vi "[Top Level] Multi Listbox.vi"() -> ()   [LabVIEW 2012]
uses:
  <vilib>/Utility/miscctls.llb/LVPoint32TypeDef.ctl
  <vilib>/Utility/error.llb/DialogType.ctl
  Method/Get Cell Item From Index.vi
  Mlistbox Tools.lvlib
panel:
  in  "Popup Listbox":i32(listbox)=4
  out "Multicolumn Listbox":i32(listbox)
  in  "Stop":bool
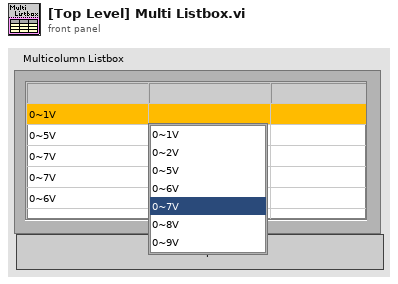
[diagram p1: front panel]
types:
  T1 = typedef "LVPoint32TypeDef.ctl" = cluster{"Horizontal":i32, "Vertical":i32}
  T2 = cluster{"State":enum16{"Initialize Multi Listbox", "Get Active Cell", "Get ItemName", "Set Symbol", "Set ItemName", "IDLE", "Error", "Exit"}, "Data":variant}
  T3 = cluster{"Multicolumn Listbox":refnum<vi>, "Popup Listbox":refnum<vi>, "Coords":T1, "Active Cell":cluster{"Row":i32, "Column":i32}, "Visible?":bool, "ItemName":string}
  T4 = enum16{"Initialize Multi Listbox", "Get Active Cell", "Get ItemName", "Set Symbol", "Set ItemName", "IDLE", "Error", "Exit"}
  T5 = cluster{"State":enum16{"Initialize Multi Listbox", "Get Active Cell", "Get ItemName", "Set Symbol", "Set ItemName", "IDLE", "Error", "Exit"}, "Data":variant}[]
  T6 = typedef "LVRowAndColumnTypeDef.ctl" = cluster{"Row":i32, "Column":i32}
  T7 = typedef "DialogType.ctl" = u16
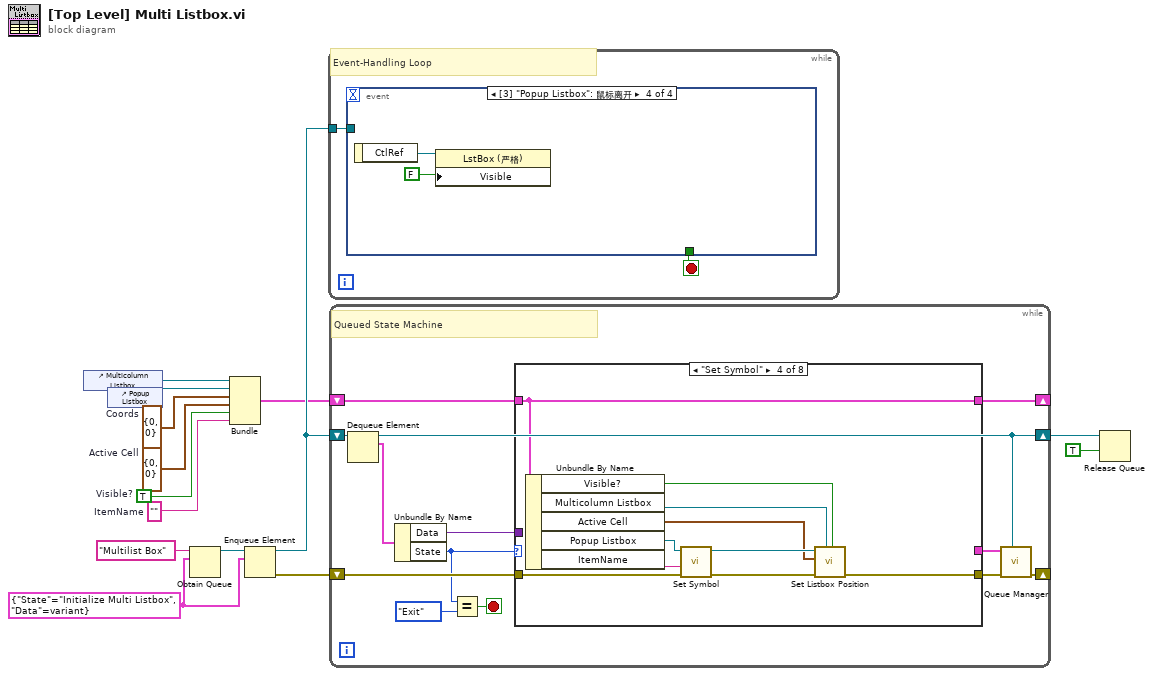
[diagram p0: block diagram]
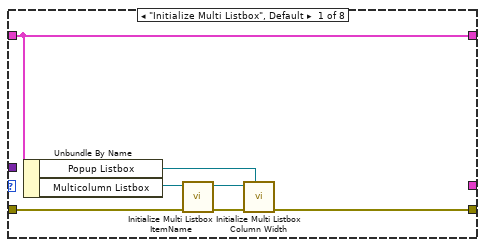
[diagram p2: hidden frame]
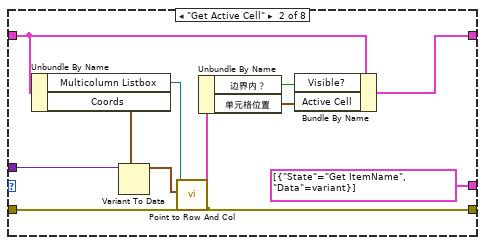
[diagram p3: hidden frame]
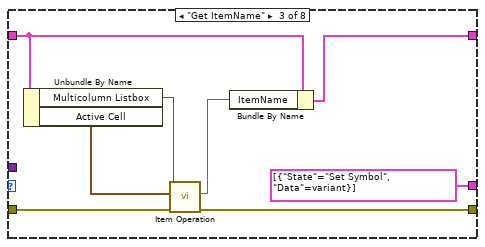
[diagram p4: hidden frame]
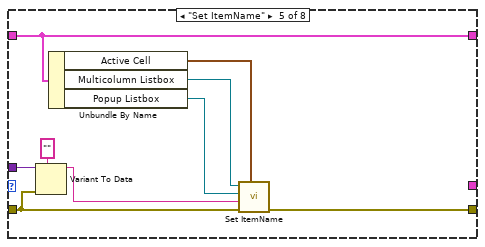
[diagram p5: hidden frame]
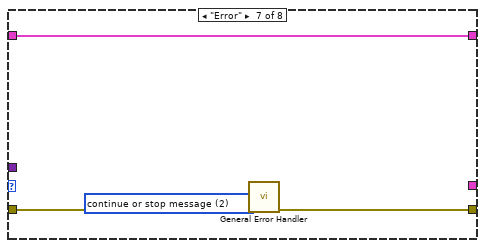
[diagram p7: hidden frame]
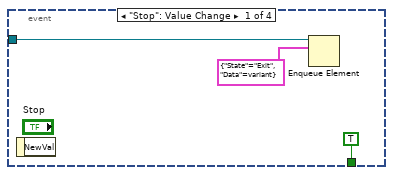
[diagram p9: hidden frame]
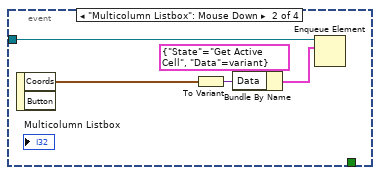
[diagram p10: hidden frame]
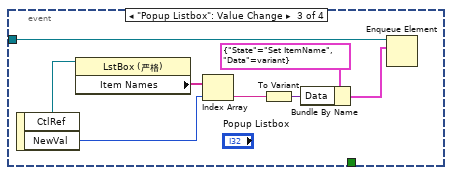
[diagram p11: hidden frame]
diagram:
  w1 = ""  # ItemName
  w2 = TRUE  # Visible?
  w3 = cluster{"Row":i32, "Column":i32} {"Row"=0, "Column"=0}  # Active Cell
  w4 = T1 {"Horizontal"=0, "Vertical"=0}  # Coords
  w8 = T2 {"State"=enum."Initialize Multi Listbox", "Data"=variant} ("Element")
  n1 = control-ref of="Multicolumn Listbox"() -> (w7:refnum<vi>)
  n2 = control-ref of="Popup Listbox"() -> (w6:refnum<vi>)
  n3 = Obtain Queue(name (unnamed)="Multilist Box", element data type=w8) -> (queue out=w10:refnum<queue>)  [unwired: 3 in, 2 out]
  n4 = Bundle ("捆绑")("Multicolumn Listbox"=w7, "Popup Listbox"=w6, "Coords"=w4, "Active Cell"=w3, "Visible?"=w2, "ItemName"=w1) -> (w5:T3)  [unwired: 1 out]
  n5 = Enqueue Element(queue=w10, element=w8) -> (queue out=w14:refnum<queue>, error out=w11:errorcluster)  [unwired: 1 in, 2 out]
  n6 = while {
    tunnel: w14 -> [w16]
    stop <- w15 stop-if-true
    # "Event-Handling Loop"
    n7 = event shown="[3] \"Popup Listbox\": 鼠标离开" {
      selector: _ -> [_ _ _ _]
      dyn-events: _ -> [_ _ _ _]
      timeout: _ -> [_ _ _ _]
      tunnel: w16 -> [w19 w24 w32 _]
      tunnel: [TRUE _ _ _] -> w15
      event "Stop": Value Change {
        n8 = event-data() -> ()  [unwired: 2 out]
        n9 = Enqueue Element(queue=w19, element=T2 {"State"=enum."Exit", "Data"=variant}) -> ()  [unwired: 1 in, 4 out]
      }
      event "Multicolumn Listbox": Mouse Down {
        n10 = event-data() -> ("Coords"=w20:T1)  [unwired: 2 out]
        n11 = To Variant(anything=w20) -> (Variant=w21:variant)
        n12 = Bundle By Name(cluster=T2 {"State"=enum."Get Active Cell", "Data"=variant} ("element"), "Data"=w21) -> (w22:T2)
        n13 = Enqueue Element(queue=w24, element=w22) -> ()  [unwired: 1 in, 4 out]
      }
      event "Popup Listbox": Value Change {
        n14 = event-data() -> ("CtlRef"=w28:refnum<vi>, "NewVal"=w26:i32)  [unwired: 1 out]
        n15 = property class="LstBox (严格)"(reference=w28) -> ("Item Names"=w27:string[])  [unwired: 1 in, 2 out]
        n16 = Index Array(array=w27, index=w26) -> (element=w25:string)
        n17 = To Variant(anything=w25) -> (Variant=w29:variant)
        n18 = Bundle By Name(cluster=T2 {"State"=enum."Set ItemName", "Data"=variant} ("element"), "Data"=w29) -> (w30:T2)
        n19 = Enqueue Element(queue=w32, element=w30) -> ()  [unwired: 1 in, 4 out]
      }
      event "Popup Listbox": Mouse Leave {
        n20 = event-data() -> ("CtlRef"=w34:refnum<vi>)  [unwired: 1 out]
        n21 = property class="LstBox (严格)"(reference=w34, "Visible"=FALSE) -> ()  [unwired: 1 in, 2 out]
      }
    }
  }
  n22 = while {
    shift-right: [w40] -> _
    shift-left: w11 -> [w44]
    shift-right: [w41] -> w12
    shift-left: w14 -> [w47]
    shift-right: [w37] -> _
    shift-left: w5 -> [w38]
    stop <- w42 stop-if-true
    # "Queued State Machine"
    n23 = Dequeue Element(queue=w47) -> (queue out=w41:refnum<queue>, element=w46:T2)  [unwired: 1 in, 3 out]
    n24 = Unbundle By Name(w46) -> ("Data"=w45:variant, "State"=w43:T4)
    n25 = Equal?(x=w43, y=T4."Exit") -> (x = y?=w42:bool)
    n26 = case shown="\"Set Symbol\"" w43 {
      tunnel: w45 -> [_ w66 _ _ w92 _ _ _]
      tunnel: w44 -> [w52 w60 w69 w82 w86 w94 w98 w100]
      tunnel: w38 -> [w54 w64 w73 w84 w93 w95 w99 w101]
      tunnel: [w54 w63 w72 w84 w93 w95 w99 w101] -> w37
      tunnel: [w48 w59 w68 w78 w85 w94 w97 w100] -> w36
      tunnel: [_ T5 [{"State"=enum."Get ItemName", "Data"=variant}] ("Elements") T5 [{"State"=enum."Set Symbol", "Data"=variant}] ("Elements") _ _ _ _ _] -> w35
      frame "Initialize Multi Listbox", Default {
        n27 = Unbundle By Name(w54) -> ("Popup Listbox"=w51:refnum<vi>, "Multicolumn Listbox"=w53:refnum<vi>)
        n28 = call "Initialize Multi Listbox ItemName.vi"("error in (no error)"=w52, "Multicolumn Listbox In"=w53) -> ("error out"=w49:errorcluster, "Multicolumn Listbox Out"=w50:refnum<vi>)  [unwired: 1 in, 7 out]
        n29 = call "Initialize Multi Listbox Column Width.vi"("Popup Listbox"=w51, "error in (no error)"=w49, "Multicolumn Listbox Out"=w50) -> ("error out"=w48:errorcluster)  [unwired: 7 out]
      }
      frame "Get Active Cell" {
        n30 = Unbundle By Name(w64) -> ("Multicolumn Listbox"=w61:refnum<vi>, "Coords"=w65:T1)
        n31 = Variant To Data(type=w65, Variant=w66) -> (data=w58:T1)  [unwired: 1 in, 1 out]
        n32 = call "Point to Row And Col.vi"("错误输入（无错误）"=w60, "点"=w58, "Ref"=w61) -> ("错误输出"=w59:errorcluster, "Point to Row and Col"=w57:cluster{"单元格位置":T6, "边界内？":bool, "符号内？":bool})  [unwired: 6 in, 1 out]
        n33 = Unbundle By Name(w57) -> ("边界内？"=w55:bool, "单元格位置"=w56:T6)
        n34 = Bundle By Name(cluster=w64, "Visible?"=w55, "Active Cell"=w56) -> (w63:T3)
      }
      frame "Get ItemName" {
        n35 = Unbundle By Name(w73) -> ("Multicolumn Listbox"=w71:refnum<vi>, "Active Cell"=w70:cluster{"Row":i32, "Column":i32})
        n36 = call-poly "Item Operation.vi"("错误输入"=w69, "Index"=w70, "Mlistbox Ref"=w71) -> ("错误输出"=w68:errorcluster, "Item"=w67:string)  [unwired: 6 in, 1 out]
        n37 = Bundle By Name(cluster=w73, "ItemName"=w67) -> (w72:T3)
      }
      frame "Set Symbol" {
        n38 = Unbundle By Name(w84) -> ("Visible?"=w75:bool, "Multicolumn Listbox"=w76:refnum<vi>, "Active Cell"=w77:cluster{"Row":i32, "Column":i32}, "Popup Listbox"=w81:refnum<vi>, "ItemName"=w83:string)
        n39 = call "Set Symbol.vi"("error in (no error)"=w82, "ItemName"=w83, "Popup Listbox In"=w81) -> ("error out"=w79:errorcluster, "Popup Listbox Out"=w80:refnum<vi>)  [unwired: 6 out]
        n40 = call "Set Listbox Position.vi"("Visible?"=w75, "Multicolumn Listbox"=w76, "error in (no error)"=w79, "Active Cell"=w77, "Popup Listbox"=w80) -> ("error out"=w78:errorcluster)  [unwired: 6 out]
      }
      frame "Set ItemName" {
        n41 = Variant To Data(error in=w86, type="" ("element"), Variant=w92) -> (data=w87:string)  [unwired: 1 out]
        n42 = Unbundle By Name(w93) -> ("Active Cell"=w89:cluster{"Row":i32, "Column":i32}, "Multicolumn Listbox"=w90:refnum<vi>, "Popup Listbox"=w88:refnum<vi>)
        n43 = call "Set ItemName.vi"("Active Cell"=w89, "error in (no error)"=w86, "ItemName"=w87, "Popup Listbox"=w88, "Multicolumn Listbox"=w90) -> ("error out"=w85:errorcluster)  [unwired: 3 in, 3 out]
      }
      frame "IDLE" {
      }
      frame "Error" {
        w96 = T7 2 items=["no dialog", "OK message", "continue or stop message", "OK message + warnings", "continue/stop + warnings"] ("type of dialog (OK msg:1)")
        n44 = call <vilib>:"General Error Handler.vi"("type of dialog (OK msg:1)"=w96, "error in (no error)"=w98) -> ("error out"=w97:errorcluster)  [unwired: 13 out]
      }
      frame "Exit" {
      }
    }
    n45 = call "Queue Manager.vi"("Queue In"=w41, "error in (no error)"=w36, "Elements"=w35) -> ("error out"=w40:errorcluster)  [unwired: 1 in, 7 out]
  }
  n46 = Release Queue(queue=w12, force destroy? (F)=TRUE) -> ()  [unwired: 1 in, 3 out]
